vi "Overall Heat Transfer Coefficient.vi"(4 "Thermal Conductivity of Hastealloy N (W/m-K)":dbl, 5 "Air Heat Xfer Coeff":dbl, 6 "Wall Thickness (m)":dbl, 7 "Sec Heat Xfer Coeff":dbl, 9 "Am":dbl, 10 "Ai":dbl, 11 "Ao":dbl) -> (3 "Overall Heat Xfer Coeff":dbl)   [LabVIEW 2019]
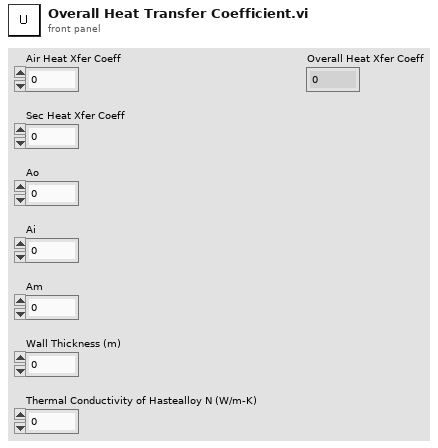
[diagram p1: front panel]
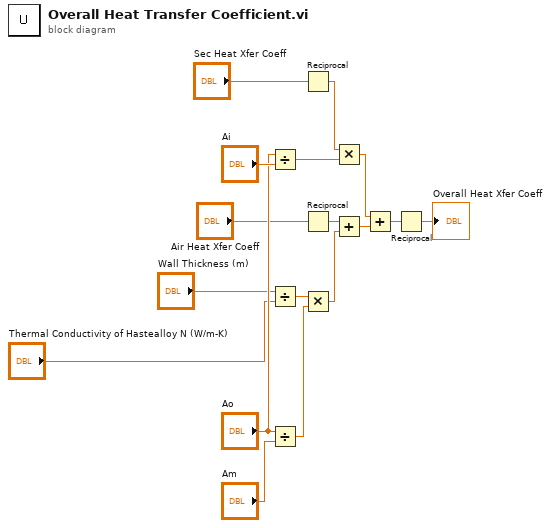
[diagram p0: block diagram]
diagram:
  n1 = Divide(x="Ao", y="Ai") -> (x/y=w11:dbl)
  n2 = Divide(x="Wall Thickness (m)", y="Thermal Conductivity of Hastealloy N (W/m-K)") -> (x/y=w5:dbl)
  n3 = Divide(x="Ao", y="Am") -> (x/y=w7:dbl)
  n4 = Reciprocal(x="Sec Heat Xfer Coeff") -> (1/x=w10:dbl)
  n5 = Reciprocal(x="Air Heat Xfer Coeff") -> (1/x=w2:dbl)
  n6 = Multiply(x=w5, y=w7) -> (x*y=w8:dbl)
  n7 = Multiply(x=w10, y=w11) -> (x*y=w14:dbl)
  n8 = Add(x=w2, y=w8) -> (x+y=w15:dbl)
  n9 = Add(x=w14, y=w15) -> (x+y=w16:dbl)
  n10 = Reciprocal(x=w16) -> (1/x=→"Overall Heat Xfer Coeff":dbl)
